vi "Shoot.vi"   [LabVIEW 2015]
uses:
  GeneralGlobals.vi
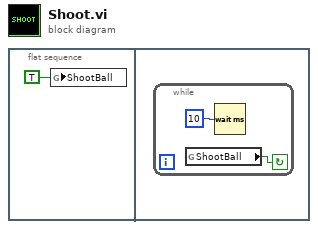
[diagram p0: block diagram]
diagram:
  n1 = flat-sequence {
    frame #0 {
      n2 = global write "GeneralGlobals.vi" "ShootBall"(TRUE ("ShootBall")) -> ()
    }
    frame #1 {
      n3 = while {
        stop <- w3 continue-if-true
        n4 = global read "GeneralGlobals.vi" "ShootBall"() -> (w3:bool)
        n5 = Wait (ms)(milliseconds to wait=u32 10) -> ()  [unwired: 1 out]
      }
    }
  }
